vi "Error Reported.vi"(8 "error in (no error)":errorcluster, 9 "Additional Information":string, 10 "Error":errorcluster, 11 "Module ID":i32=-1) -> (0 "error out":errorcluster)   [LabVIEW 2014, in "Configurable.lvlib"]
doc: "Send the Error Reported event to any VI registered to listen to events from the owning module.\n_____\nBased on Delacor QMH Project Template 4.0.0.47."
uses:
  Configurable.lvlib
  Error Reported Argument--cluster.ctl
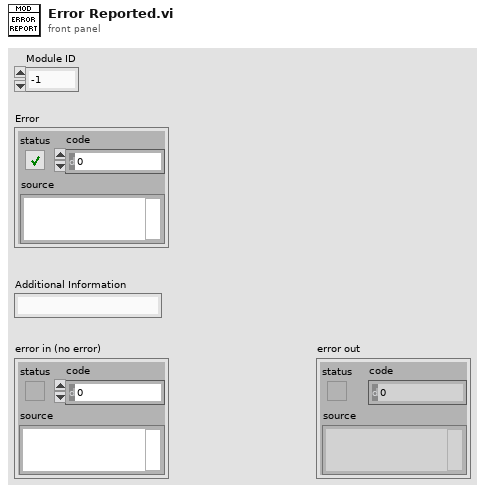
[diagram p1: front panel]
types:
  T1 = typedef "Configurable.lvlib/Error Reported Argument--cluster.ctl" = cluster{"Error":errorcluster, "Additional Information":string, "Module ID":i32, "Module Name":string}
  T2 = typedef "Configurable.lvlib/Broadcast Events--cluster.ctl" = cluster{"Module Did Init":refnum<user-event>, "Status Updated":refnum<user-event>, "Error Reported":refnum<user-event>, "Module Did Stop":refnum<user-event>, "Update Module Execution Status":refnum<user-event>}
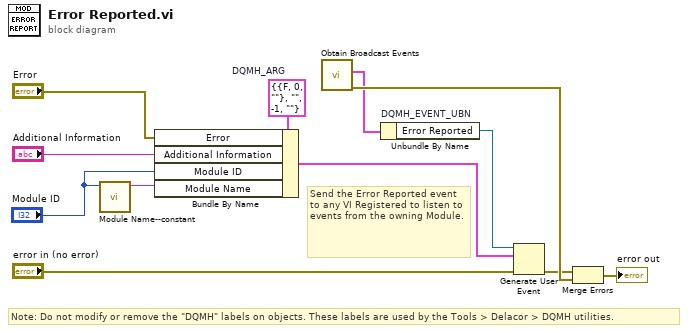
[diagram p0: block diagram]
diagram:
  w5 = T1 {"Error"={"status"=FALSE, "code"=0, "source"=""}, "Additional Information"="", "Module ID"=-1, "Module Name"=""}  # DQMH_ARG
  # "Note: Do not modify or remove the \"DQMH\" labels on objects. These labels are used by the Tools > Delacor > DQMH utilities."
  # "Send the Error Reported event to any VI Registered to listen to events from the owning Module."
  n1 = call "Module Name--constant.vi"("Module ID"="Module ID") -> ("Module Name"=w1:string)  [unwired: 10 in]
  n2 = Bundle By Name(cluster=w5, "Error"="Error", "Additional Information"="Additional Information", "Module ID"="Module ID", "Module Name"=w1) -> (w4:T1)
  n3 = call "Obtain Broadcast Events.vi"() -> ("error out"=w9:errorcluster, "Configurable Broadcast Events"=w7:T2)  [unwired: 10 in]
  n4 = Unbundle By Name "DQMH_EVENT_UBN"(w7) -> ("Error Reported"=w6:refnum<user-event>)
  n5 = Generate User Event(user event=w6, event data cluster=w4, error in="error in (no error)") -> (error out=w8:errorcluster)  [unwired: 1 in, 1 out]
  n6 = Merge Errors(w8, w9) -> (→"error out":errorcluster)
